vi "Poly_Text_Write.vi"(5 "File Position":enum16{"start", "end", "current"}(ring)=enum."current", 6 "Auto Increment":bool, 7 "Text":string, 8 "error in":errorcluster, 9 "access (0:read/write)":enum16{"read/write", "read-only", "write-only"}(ring), 10 "operation (0:open)":T1(ring)=enum."open or create", 11 "file path":path) -> (0 "error out":errorcluster)   [LabVIEW 2024, in "Launcher_DTU.lvlib"]
uses:
  Launcher_DTU.lvlib
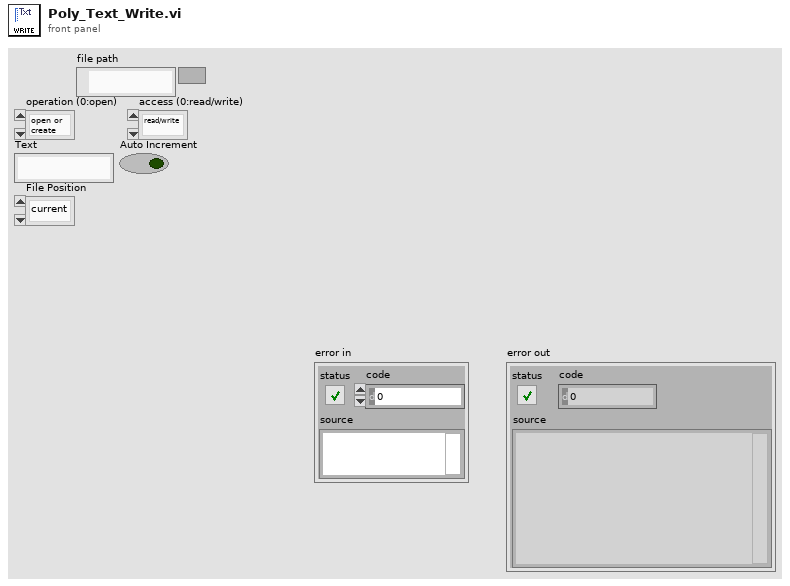
[diagram p1: front panel]
types:
  T1 = enum16{"open", "replace", "create", "open or create", "replace or create", "replace or create with confirmation"}
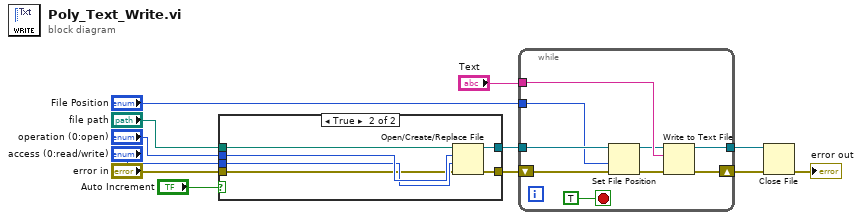
[diagram p0: block diagram]
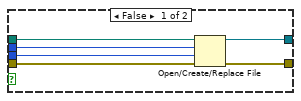
[diagram p2: hidden frame]
diagram:
  n1 = case shown="True" "Auto Increment" {
    tunnel: "error in" -> [w18 w20]
    tunnel: [w17 w24] -> w10
    tunnel: "file path" -> [w16 w19]
    tunnel: "operation (0:open)" -> [w15 w22]
    tunnel: "access (0:read/write)" -> [w14 w21]
    tunnel: [w13 w23] -> w6
    frame False {
      n2 = Open/Create/Replace File(file path (use dialog)=w16, error in=w18, operation (0:open)=w15, access (0:read/write)=w14) -> (refnum out=w13:refnum<file>, error out=w17:errorcluster)  [unwired: 2 in, 1 out]
    }
    frame True {
      n3 = Open/Create/Replace File(file path (use dialog)=w19, error in=w20, operation (0:open)=w22, access (0:read/write)=w21) -> (refnum out=w23:refnum<file>, error out=w24:errorcluster)  [unwired: 2 in, 1 out]
    }
  }
  n4 = while {
    shift-right: [w32] -> w11
    shift-left: w10 -> [w29]
    tunnel: w6 -> [w27]
    tunnel: "Text" -> [w31]
    tunnel: [w30] -> w3
    tunnel: "File Position" -> [w25]
    stop <- TRUE stop-if-true
    n5 = Set File Position(refnum=w27, from (0:start)=w25, error in=w29) -> (refnum out=w26:refnum<file>, error out=w28:errorcluster)  [unwired: 1 in]
    n6 = Write to Text File(file (use dialog)=w26, text=w31, error in=w28) -> (refnum out=w30:refnum<file>, error out=w32:errorcluster)  [unwired: 1 in, 1 out]
  }
  n7 = Close File(refnum=w3, error in=w11) -> (error out=→"error out":errorcluster)  [unwired: 1 out]
